vi "Begin.vi"(8 "error in":errorcluster) -> (0 "error out":errorcluster)   [LabVIEW 2015]
doc: "Called before other user functions, this VI is expected to open initial I/O refnums, load in file data, and do all program initialization. Notice that the <B>error out</B> terminal is simply used for data flow. Wiring it to other structures or subVIs ensures that this VI runs first."
uses:
  <vilib>/Rock Robotics/WPI/DriverStation/WPI_DriverStationRobotMode2.ctl
  <vilib>/Rock Robotics/WPI/Joystick/WPI_JoystickDeviceEnum.ctl
  <vilib>/Rock Robotics/WPI/Solenoid/WPI_SolenoidChannel.ctl
  <vilib>/Rock Robotics/WPI/CAN/TalonSRX/WPI_CANTalonSRX_BrakeOverride.ctl
  <vilib>/Rock Robotics/WPI/CAN/TalonSRX/WPI_CANTalonSRX_APIControlMode.ctl
  <vilib>/Rock Robotics/SystemInterfaces/DIO/FPGA_DIOChannel.ctl
  <vilib>/Rock Robotics/WPI/Camera/WPI_CameraWhite Balance Values.ctl
  <vilib>/Rock Robotics/WPI/Camera/WPI_CameraExposure Values.ctl
  Robot Global Data.vi
  <vilib>/Rock Robotics/WPI/Utilities/WPI_GetSetVariantRefNum.vi
  <vilib>/Rock Robotics/WPI/Solenoid/WPI_SolenoidOpenSingle.vi
  <vilib>/Rock Robotics/WPI/MotorControl/WPI_MotorControlOpenCANTalonSRX.vi
  <vilib>/Rock Robotics/SystemInterfaces/DIO/FPGA_DIOPWMChannel.ctl
  <vilib>/Rock Robotics/Network Tables/NT Write String Array.vi
  <vilib>/Rock Robotics/WPI/Counter/WPI_CounterDigitalInputToDigitalSource.vi
  <vilib>/Rock Robotics/WPI/RobotDrive/WPI_RobotDriveOpen2MotorWithTalon.vi
  <vilib>/Rock Robotics/WPI/SafetyOutput/WPI_SafetyOutputConfigMenu.ctl
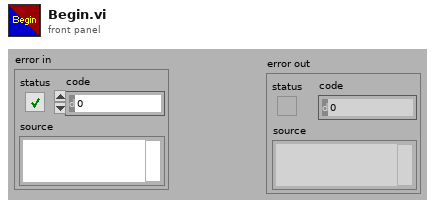
[diagram p1: front panel]
types:
  T1 = typedef "WPI_CANTalonSRX_BrakeOverride.ctl" = enum8{"No Override", "Override to Coast", "Override to Brake"}
  T2 = typedef "FPGA_DIOChannel.ctl" = enum8{"DIO 0", "DIO 1", "DIO 2", "DIO 3", "DIO 4", "DIO 5", "DIO 6", "DIO 7", "DIO 8", "DIO 9", "DIO MXP 0", "DIO MXP 1", "DIO MXP 2", "DIO MXP 3", "DIO MXP 4", "DIO MXP 5", "DIO MXP 6", "DIO MXP 7", "DIO MXP 8", "DIO MXP 9", "DIO MXP 10", "DIO MXP 11", "DIO MXP 12", "DIO MXP 13", "DIO MXP 14", "DIO MXP 15", "Invalid"}
  T3 = typedef "WPI_JoystickDeviceEnum.ctl" = enum16{"USB 0", "USB 1", "USB 2", "USB 3", "USB 4", "USB 5"}
  T4 = typedef "WPI_SolenoidChannel.ctl" = enum8{"Solenoid 0", "Solenoid 1", "Solenoid 2", "Solenoid 3", "Solenoid 4", "Solenoid 5", "Solenoid 6", "Solenoid 7", "Invalid"}
  T5 = typedef "WPI_CANTalonSRX_APIControlMode.ctl" = enum8{"Percent VBus", "Speed", "Position", "Slave", "Unchanged / Invalid", "Voltage Compensation", "Current", "Motion Profile"}
  T6 = typedef "WPI_DriverStationRobotMode2.ctl" = enum16{"Autonomous Disabled", "Autonomous Enabled", "Teleop Disabled", "Teleop Enabled", "Disconnected", "Finish", "Test Disabled", "Test Enabled", "Emergency Stopped"}
  T7 = typedef "WPI_CameraExposure Values.ctl" = enum16{"Auto", "Flicker-free 50 Hz", "Flicker-free 60 Hz", "Hold current", "Custom"}
  T8 = typedef "WPI_CameraWhite Balance Values.ctl" = enum16{"Auto", "Fixed indoor", "Fixed outdoor 1", "Fixed outdoor 2", "Fixed fluorescent 1", "Fixed fluorescent 2", "Hold current", "Custom"}
  T9 = typedef "WPI_CameraDevRef.ctl" = cluster{"Camera Address":string, "CameraStatus":errorcluster}
  T10 = typedef "WPI_DigitalInputDevRef.ctl" = cluster{"DevStatus":errorcluster, "DIO Channel":T2}
  T11 = typedef "FPGA_CounterEncoderSourceConvertionLVSourceType.ctl" = cluster{"DevStatus":errorcluster, "AnalogTriggerMode?":bool, "DigitalMode":cluster{"DIO Channel":T12}, "AnalogTriggerMode":cluster{"AnalogTriggerIndex":T13, "OutputType":T14}}
  T12 = typedef "FPGA_DIODigitalSourceChannel.ctl" = enum8{"DIO 0", "DIO 1", "DIO 2", "DIO 3", "DIO 4", "DIO 5", "DIO 6", "DIO 7", "DIO 8", "DIO 9", "DIO MXP 0", "DIO MXP 1", "DIO MXP 2", "DIO MXP 3", "DIO MXP 4", "DIO MXP 5", "DIO MXP 6", "DIO MXP 7", "DIO MXP 8", "DIO MXP 9", "DIO MXP 10", "DIO MXP 11", "DIO MXP 12", "DIO MXP 13", "DIO MXP 14", "DIO MXP 15", "Disabled"}
  T13 = typedef "FPGA_AnalogTriggerIndex.ctl" = enum8{"Trig 0", "Trig 1", "Trig 2", "Trig 3", "Trig 4", "Trig 5", "Trig 6", "Trig 7", "Invalid"}
  T14 = typedef "FPGA_AnalogTriggerOutType.ctl" = enum16{"InWindow", "TriggerState", "Rising", "Falling"}
  T15 = typedef "WPI_EncoderDevRef.ctl" = cluster{"DevStatus":errorcluster, "EncoderIndex":T16, "CounterIndex":T17, "DistancePerCount":dbl, "Decoding Type":T18}
  T16 = typedef "FPGA_EncoderIdx.ctl" = enum8{"Enc 0", "Enc 1", "Enc 2", "Enc 3", "Enc 4", "Enc 5", "Enc 6", "Enc 7", "Invalid"}
  T17 = typedef "FPGA_CounterCtrSystemIndex.ctl" = enum8{"Ctr 0", "Ctr 1", "Ctr 2", "Ctr 3", "Ctr 4", "Ctr 5", "Ctr 6", "Ctr 7", "Invalid"}
  T18 = typedef "WPI_EncoderType.ctl" = enum16{"1x", "2x", "4x"}
  T19 = typedef "WPI_SafetyOutputConfigMenu.ctl" = enum16{"Enable", "Disable"}
  T20 = typedef "FPGA_DIOPWMChannel.ctl" = enum8{"PWM 0", "PWM 1", "PWM 2", "PWM 3", "PWM 4", "PWM 5", "PWM 6", "PWM 7", "PWM 8", "PWM 9", "PWM MXP 0", "PWM MXP 1", "PWM MXP 2", "PWM MXP 3", "PWM MXP 4", "PWM MXP 5", "PWM MXP 6", "PWM MXP 7", "PWM MXP 8", "PWM MXP 9", "Invalid"}
  T21 = typedef "WPI_RobotDriveDevRef.ctl" = cluster{"DevStatus":errorcluster, "Motors[]":T22[], "Square Inputs":bool, "Max Output":dbl}
  T22 = typedef "WPI_MotorControlDeviceRef.ctl" = cluster{"DeviceStatus":errorcluster, "Type":T23, "PWM":cluster{"PWM Channel":T20, "DeadBand":T24}, "CAN":cluster{"Device Number":u8, "Control Mode":T25, "Semaphore":T26, "Max Vout":dbl, "TalonSRX Control Mode":T5}, "Invert":bool}
  T23 = typedef "WPI_MotorControlType.ctl" = enum16{"PWM", "CAN", "CANTalonSRX"}
  T24 = typedef "WPI_PWMDeadband.ctl" = cluster{"Name":string, "maxPositivePwm":i32, "minPositivePwm":i32, "centerPwm":i32, "maxNegativePwm":i32, "minNegativePwm":i32, "angularRange":u16}
  T25 = typedef "WPI_CANJaguar_ControlMode.ctl" = enum8{"Percent VBus", "Current", "Speed", "Position", "Voltage"}
  T26 = typedef "Semaphore RefNum" = refnum<k1>
  T27 = typedef "WPI_SolenoidDevRef.ctl" = cluster{"DevStatus":errorcluster, "Pneumatics Control Module":u8, "Forward Solenoid Channel":T4, "Reverse Solenoid Channel":T4}
  T28 = typedef "WPI_CompressorDevRef.ctl" = cluster{"DevStatus":errorcluster, "Pneumatics Control Module":u8}
  T29 = typedef "WPI_JoystickDevRef.ctl" = cluster{"Device":T3}
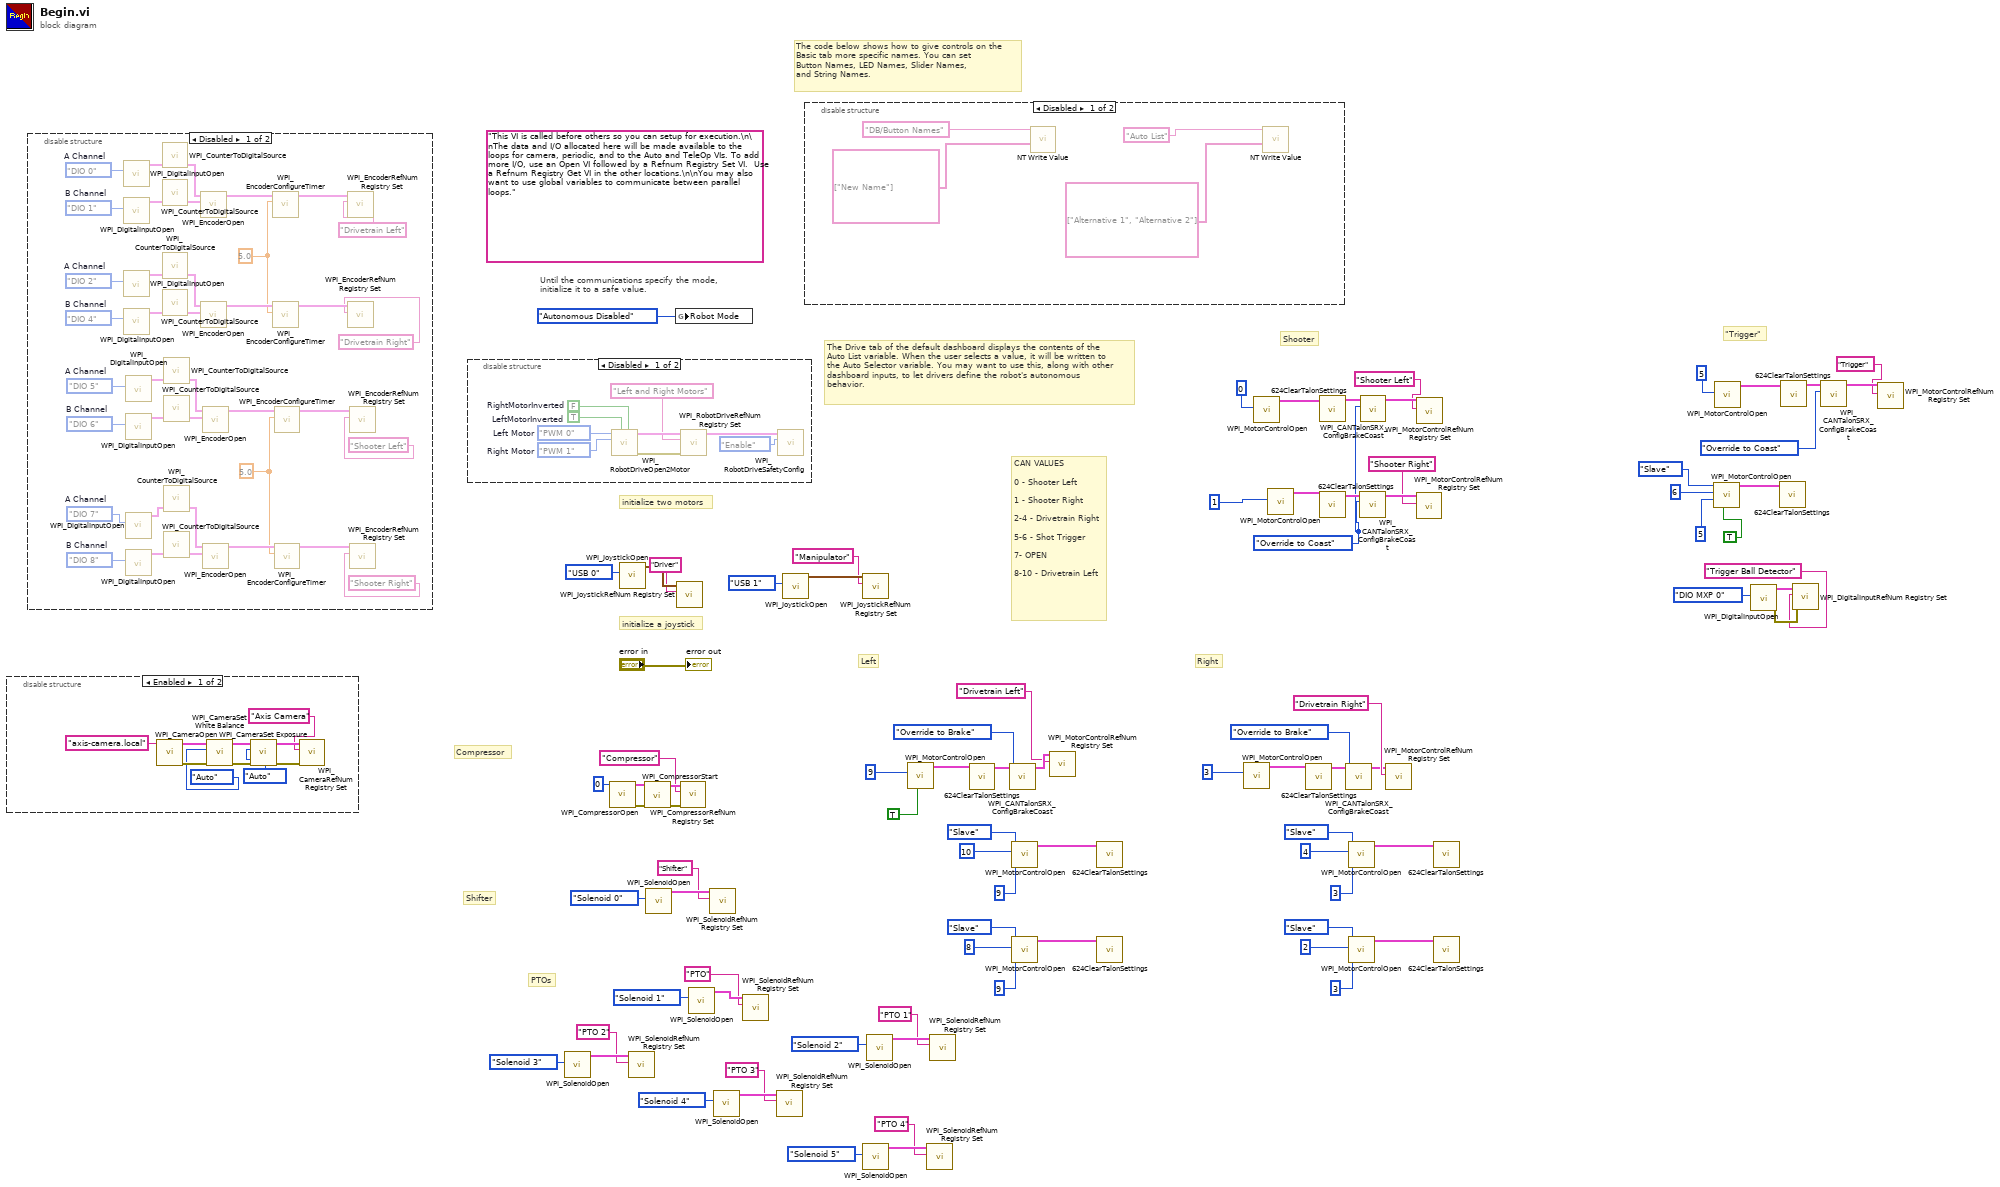
[diagram p0: block diagram]
diagram:
  w42 = WPI_CANTalonSRX_BrakeOverride."Override to Coast" ("Brake / Coast Mode")
  (unwired) "This VI is called before others so you can setup for execution.\n\nThe data and I/O allocated here will be made available to the loops for camera, periodic, and to the Auto and TeleOp VIs. To add more I/O, use an Open VI followed by a Refnum Registry Set VI.  Use a Refnum Registry Get VI in the other locations.\n\nYou may also want to use global variables to communicate between parallel loops."
  # "\"Trigger\""
  # "CAN VALUES\n\n0 - Shooter Left\n\n1 - Shooter Right\n\n2-4 - Drivetrain Right\n\n5-6 - Shot Trigger\n\n7- OPEN\n\n8-10 - Drivetrain Left"
  # "PTOs"
  # "Shooter"
  # "Left"
  # "Right"
  # "Shifter"
  # "Compressor"
  # "The Drive tab of the default dashboard displays the contents of the\nAuto List variable. When the user selects a value, it will be written to\nthe Auto Selector variable. You may want to use this, along with other\ndashboard inputs, to let drivers define the robot's autonomous\nbehavior."
  # "The code below shows how to give controls on the\nBasic tab more specific names. You can set\nButton Names, LED Names, Slider Names,\nand String Names."
  # "initialize a joystick"
  # "Until the communications specify the mode,\ninitialize it to a safe value."
  # "initialize two motors"
  n1 = disable-structure shown="Enabled" {
    frame Enabled {
      n2 = call <vilib>:"WPI_CameraOpen.vi"("Camera Address"="axis-camera.local") -> ("error out"=w93:errorcluster, "CameraDevRef"=w92:T9)  [unwired: 9 in]
      n3 = call <vilib>:"WPI_CameraSet White Balance.vi"("error in (no error)"=w93, "White Balance"=WPI_CameraWhite_Balance_Values."Auto", "CameraDevRef"=w92) -> ("error out"=w95:errorcluster, "CameraDevRef Out"=w94:T9)  [unwired: 7 in]
      n4 = call <vilib>:"WPI_CameraSet Exposure.vi"("error in (no error)"=w95, "Exposure"=WPI_CameraExposure_Values."Auto", "CameraDevRef"=w94) -> ("error out"=w97:errorcluster, "CameraDevRef Out"=w96:T9)  [unwired: 7 in]
      n5 = call <vilib>:"WPI_CameraRefNum Registry Set.vi"("error in (no error)"=w97, "refnum name"="Axis Camera", "CameraDevRef"=w96) -> ()  [unwired: 7 in, 2 out]
    }
    frame Disabled {
    }
  }
  n6 = disable-structure shown="Disabled" {
    frame Disabled {
      w100 = FPGA_DIOChannel."DIO 0"  # A Channel
      w103 = FPGA_DIOChannel."DIO 1"  # B Channel
      w108 = 5.0 ("Minimum Rate")
      w109 = FPGA_DIOChannel."DIO 2"  # A Channel
      w112 = FPGA_DIOChannel."DIO 4"  # B Channel
      w119 = FPGA_DIOChannel."DIO 6"  # B Channel
      w122 = FPGA_DIOChannel."DIO 5"  # A Channel
      w127 = 5.0 ("Minimum Rate")
      w128 = FPGA_DIOChannel."DIO 8"  # B Channel
      w131 = FPGA_DIOChannel."DIO 7"  # A Channel
      n7 = call <vilib>:"WPI_DigitalInputOpen.vi"("DIO Channel"=w100) -> ("DigitalInputDevRef"=w101:T10)  [unwired: 1 in, 9 out]
      n8 = call <vilib>:"WPI_DigitalInputOpen.vi"("DIO Channel"=w103) -> ("DigitalInputDevRef"=w104:T10)  [unwired: 1 in, 9 out]
      n9 = call <vilib>:"WPI_DigitalInputOpen.vi"("DIO Channel"=w109) -> ("DigitalInputDevRef"=w110:T10)  [unwired: 1 in, 9 out]
      n10 = call <vilib>:"WPI_DigitalInputOpen.vi"("DIO Channel"=w112) -> ("DigitalInputDevRef"=w113:T10)  [unwired: 1 in, 9 out]
      n11 = call <vilib>:"WPI_DigitalInputOpen.vi"("DIO Channel"=w122) -> ("DigitalInputDevRef"=w123:T10)  [unwired: 1 in, 9 out]
      n12 = call <vilib>:"WPI_DigitalInputOpen.vi"("DIO Channel"=w119) -> ("DigitalInputDevRef"=w120:T10)  [unwired: 1 in, 9 out]
      n13 = call <vilib>:"WPI_DigitalInputOpen.vi"("DIO Channel"=w131) -> ("DigitalInputDevRef"=w132:T10)  [unwired: 1 in, 9 out]
      n14 = call <vilib>:"WPI_DigitalInputOpen.vi"("DIO Channel"=w128) -> ("DigitalInputDevRef"=w129:T10)  [unwired: 1 in, 9 out]
      n15 = call-poly <vilib>:"WPI_CounterToDigitalSource.vi"("DigitalInputDevRef"=w101) -> ("Digital Source"=w102:T11)  [unwired: 6 out]
      n16 = call-poly <vilib>:"WPI_CounterToDigitalSource.vi"("DigitalInputDevRef"=w104) -> ("Digital Source"=w105:T11)  [unwired: 6 out]
      n17 = call-poly <vilib>:"WPI_CounterToDigitalSource.vi"("DigitalInputDevRef"=w110) -> ("Digital Source"=w111:T11)  [unwired: 6 out]
      n18 = call-poly <vilib>:"WPI_CounterToDigitalSource.vi"("DigitalInputDevRef"=w113) -> ("Digital Source"=w114:T11)  [unwired: 6 out]
      n19 = call-poly <vilib>:"WPI_CounterToDigitalSource.vi"("DigitalInputDevRef"=w123) -> ("Digital Source"=w124:T11)  [unwired: 6 out]
      n20 = call-poly <vilib>:"WPI_CounterToDigitalSource.vi"("DigitalInputDevRef"=w120) -> ("Digital Source"=w121:T11)  [unwired: 6 out]
      n21 = call-poly <vilib>:"WPI_CounterToDigitalSource.vi"("DigitalInputDevRef"=w132) -> ("Digital Source"=w133:T11)  [unwired: 6 out]
      n22 = call-poly <vilib>:"WPI_CounterToDigitalSource.vi"("DigitalInputDevRef"=w129) -> ("Digital Source"=w130:T11)  [unwired: 6 out]
      n23 = call <vilib>:"WPI_EncoderOpen.vi"("BSource"=w105, "ASource"=w102) -> ("EncoderDevRef"=w106:T15)  [unwired: 6 in, 3 out]
      n24 = call <vilib>:"WPI_EncoderOpen.vi"("BSource"=w114, "ASource"=w111) -> ("EncoderDevRef"=w115:T15)  [unwired: 6 in, 3 out]
      n25 = call <vilib>:"WPI_EncoderOpen.vi"("BSource"=w121, "ASource"=w124) -> ("EncoderDevRef"=w125:T15)  [unwired: 6 in, 3 out]
      n26 = call <vilib>:"WPI_EncoderOpen.vi"("BSource"=w130, "ASource"=w133) -> ("EncoderDevRef"=w134:T15)  [unwired: 6 in, 3 out]
      n27 = call <vilib>:"WPI_EncoderConfigureTimer.vi"("Minimum Rate"=w108, "EncoderDevRef"=w106) -> ("EncoderDevRef"=w107:T15)  [unwired: 8 in, 1 out]
      n28 = call <vilib>:"WPI_EncoderConfigureTimer.vi"("Minimum Rate"=w108, "EncoderDevRef"=w115) -> ("EncoderDevRef"=w116:T15)  [unwired: 8 in, 1 out]
      n29 = call <vilib>:"WPI_EncoderConfigureTimer.vi"("Minimum Rate"=w127, "EncoderDevRef"=w125) -> ("EncoderDevRef"=w126:T15)  [unwired: 8 in, 1 out]
      n30 = call <vilib>:"WPI_EncoderConfigureTimer.vi"("Minimum Rate"=w127, "EncoderDevRef"=w134) -> ("EncoderDevRef"=w135:T15)  [unwired: 8 in, 1 out]
      n31 = call <vilib>:"WPI_EncoderRefNum Registry Set.vi"("refnum name"="Drivetrain Left", "EncoderDevRef"=w107) -> ()  [unwired: 8 in, 2 out]
      n32 = call <vilib>:"WPI_EncoderRefNum Registry Set.vi"("refnum name"="Drivetrain Right", "EncoderDevRef"=w116) -> ()  [unwired: 8 in, 2 out]
      n33 = call <vilib>:"WPI_EncoderRefNum Registry Set.vi"("refnum name"="Shooter Left", "EncoderDevRef"=w126) -> ()  [unwired: 8 in, 2 out]
      n34 = call <vilib>:"WPI_EncoderRefNum Registry Set.vi"("refnum name"="Shooter Right", "EncoderDevRef"=w135) -> ()  [unwired: 8 in, 2 out]
    }
    frame Enabled {
    }
  }
  n35 = disable-structure shown="Disabled" {
    frame Disabled {
      w138 = FPGA_DIOPWMChannel."PWM 1"  # Right Motor
      w139 = TRUE  # LeftMotorInverted
      w140 = FPGA_DIOPWMChannel."PWM 0"  # Left Motor
      w141 = FALSE  # RightMotorInverted
      n36 = call-poly <vilib>:"WPI_RobotDriveOpen2Motor.vi"("Right Motor Inverted"=w141, "Left Motor Inverted"=w139, "Right Motor"=w138, "Left Motor"=w140) -> ("error out"=w143:errorcluster, "RobotDriveDevRef"=w142:T21)  [unwired: 1 in, 5 out]
      n37 = call <vilib>:"WPI_RobotDriveRefNum Registry Set.vi"("error in (no error)"=w143, "refnum name"="Left and Right Motors", "RobotDriveDevRef"=w142) -> ("RobotDriveDevRef"=w144:T21)  [unwired: 1 in, 7 out]
      n38 = call <vilib>:"WPI_RobotDriveSafetyConfig.vi"("mode"=WPI_SafetyOutputConfigMenu."Enable", "RobotDriveDevRef"=w144) -> ()  [unwired: 8 in, 2 out]
    }
    frame Enabled {
    }
  }
  n39 = call-poly <vilib>:"WPI_SolenoidOpen.vi"("Solenoid Channel"=WPI_SolenoidChannel."Solenoid 3") -> ("SolenoidDevRef"=w27:T27)  [unwired: 9 in, 1 out]
  n40 = call <vilib>:"WPI_CompressorOpen.vi"("Pneumatics Control Module (0)"=0) -> ("CompressorDevRef"=w82:T28, "error out"=w79:errorcluster)  [unwired: 13 in]
  n41 = call <vilib>:"WPI_JoystickOpen.vi"("JoystickDevice"=WPI_JoystickDeviceEnum."USB 0") -> ("JoystickDevRef"=w86:T29)  [unwired: 10 in]
  n42 = call <vilib>:"WPI_SolenoidRefNum Registry Set.vi"("refnum name"="PTO 2", "SolenoidDevRef"=w27) -> ()  [unwired: 8 in, 2 out]
  n43 = call <vilib>:"WPI_CompressorStart.vi"("error in (no error)"=w79, "CompressorDevRef"=w82) -> ("error out"=w78:errorcluster, "CompressorDevRef"=w81:T28)  [unwired: 8 in]
  n44 = call-poly <vilib>:"WPI_SolenoidOpen.vi"("Solenoid Channel"=WPI_SolenoidChannel."Solenoid 0") -> ("SolenoidDevRef"=w76:T27)  [unwired: 9 in, 1 out]
  n45 = global write "Robot Global Data.vi" "Robot Mode"(WPI_DriverStationRobotMode2."Autonomous Disabled" ("Robot Mode")) -> ()
  n46 = call <vilib>:"WPI_JoystickRefNum Registry Set.vi"("refnum name"="Driver", "JoystickDevRef"=w86) -> ()  [unwired: 8 in, 2 out]
  n47 = call <vilib>:"WPI_CompressorRefNum Registry Set.vi"("error in (no error)"=w78, "refnum name"="Compressor", "CompressorDevRef"=w81) -> ()  [unwired: 7 in, 2 out]
  n48 = call-poly <vilib>:"WPI_SolenoidOpen.vi"("Solenoid Channel"=WPI_SolenoidChannel."Solenoid 1") -> ("SolenoidDevRef"=w35:T27)  [unwired: 9 in, 1 out]
  n49 = call <vilib>:"WPI_SolenoidRefNum Registry Set.vi"("refnum name"="Shifter", "SolenoidDevRef"=w76) -> ()  [unwired: 8 in, 2 out]
  n50 = call-poly <vilib>:"WPI_SolenoidOpen.vi"("Solenoid Channel"=WPI_SolenoidChannel."Solenoid 4") -> ("SolenoidDevRef"=w30:T27)  [unwired: 9 in, 1 out]
  n51 = call <vilib>:"WPI_SolenoidRefNum Registry Set.vi"("refnum name"="PTO", "SolenoidDevRef"=w35) -> ()  [unwired: 8 in, 2 out]
  n52 = call <vilib>:"WPI_SolenoidRefNum Registry Set.vi"("refnum name"="PTO 3", "SolenoidDevRef"=w30) -> ()  [unwired: 8 in, 2 out]
  n53 = call <vilib>:"WPI_JoystickOpen.vi"("JoystickDevice"=WPI_JoystickDeviceEnum."USB 1") -> ("JoystickDevRef"=w21:T29)  [unwired: 10 in]
  n54 = disable-structure shown="Disabled" {
    frame Disabled {
      n55 = call-poly <vilib>:"NT Write Value.vi"("String Array"=string[] ["New Name"], "Name"="DB/Button Names") -> ()  [unwired: 9 in, 1 out]
      n56 = call-poly <vilib>:"NT Write Value.vi"("String Array"=string[] ["Alternative 1", "Alternative 2"], "Name"="Auto List") -> ()  [unwired: 9 in, 1 out]
    }
    frame Enabled {
    }
  }
  n57 = call <vilib>:"WPI_JoystickRefNum Registry Set.vi"("refnum name"="Manipulator", "JoystickDevRef"=w21) -> ()  [unwired: 8 in, 2 out]
  n58 = call-poly <vilib>:"WPI_SolenoidOpen.vi"("Solenoid Channel"=WPI_SolenoidChannel."Solenoid 5") -> ("SolenoidDevRef"=w24:T27)  [unwired: 9 in, 1 out]
  n59 = call-poly <vilib>:"WPI_SolenoidOpen.vi"("Solenoid Channel"=WPI_SolenoidChannel."Solenoid 2") -> ("SolenoidDevRef"=w33:T27)  [unwired: 9 in, 1 out]
  n60 = call-poly <vilib>:"WPI_MotorControlOpen.vi"("Invert"=TRUE, "Device Number"=9) -> ("MotorControlDeviceRef"=w50:T22)  [unwired: 8 in, 1 out]
  n61 = call <vilib>:"WPI_SolenoidRefNum Registry Set.vi"("refnum name"="PTO 4", "SolenoidDevRef"=w24) -> ()  [unwired: 8 in, 2 out]
  n62 = call <vilib>:"WPI_SolenoidRefNum Registry Set.vi"("refnum name"="PTO 1", "SolenoidDevRef"=w33) -> ()  [unwired: 8 in, 2 out]
  n63 = call "624ClearTalonSettings.vi"("CAN Talon SRX Ref Out"=w50) -> ("CAN Talon SRX Ref Out 2"=w51:T22)  [unwired: 10 in]
  n64 = call <vilib>:"WPI_CANTalonSRX_ConfigBrakeCoast.vi"("Brake / Coast Mode"=WPI_CANTalonSRX_BrakeOverride."Override to Brake", "CAN Talon SRX Ref"=w51) -> ("CAN Talon SRX Ref"=w52:T22)  [unwired: 8 in, 1 out]
  n65 = call-poly <vilib>:"WPI_MotorControlOpen.vi"("Master Device Number"=u8 9, "Device Number"=u8 10, "Control Mode"=WPI_CANTalonSRX_APIControlMode."Slave") -> ("MotorControlDeviceRef"=w56:T22)  [unwired: 7 in, 1 out]
  n66 = call-poly <vilib>:"WPI_MotorControlOpen.vi"("Master Device Number"=u8 9, "Device Number"=u8 8, "Control Mode"=WPI_CANTalonSRX_APIControlMode."Slave") -> ("MotorControlDeviceRef"=w57:T22)  [unwired: 7 in, 1 out]
  n67 = call <vilib>:"WPI_MotorControlRefNum Registry Set.vi"("refnum name"="Drivetrain Left", "MotorControlDevRef"=w52) -> ()  [unwired: 8 in, 2 out]
  n68 = call "624ClearTalonSettings.vi"("CAN Talon SRX Ref Out"=w56) -> ()  [unwired: 10 in, 1 out]
  n69 = call "624ClearTalonSettings.vi"("CAN Talon SRX Ref Out"=w57) -> ()  [unwired: 10 in, 1 out]
  n70 = call-poly <vilib>:"WPI_MotorControlOpen.vi"("Device Number"=3) -> ("MotorControlDeviceRef"=w71:T22)  [unwired: 9 in, 1 out]
  n71 = call-poly <vilib>:"WPI_MotorControlOpen.vi"("Device Number"=u8 0) -> ("MotorControlDeviceRef"=w39:T22)  [unwired: 9 in, 1 out]
  n72 = call-poly <vilib>:"WPI_MotorControlOpen.vi"("Device Number"=u8 1) -> ("MotorControlDeviceRef"=w44:T22)  [unwired: 9 in, 1 out]
  n73 = call "624ClearTalonSettings.vi"("CAN Talon SRX Ref Out"=w71) -> ("CAN Talon SRX Ref Out 2"=w70:T22)  [unwired: 10 in]
  n74 = call "624ClearTalonSettings.vi"("CAN Talon SRX Ref Out"=w44) -> ("CAN Talon SRX Ref Out 2"=w45:T22)  [unwired: 10 in]
  n75 = call "624ClearTalonSettings.vi"("CAN Talon SRX Ref Out"=w39) -> ("CAN Talon SRX Ref Out 2"=w40:T22)  [unwired: 10 in]
  n76 = call <vilib>:"WPI_CANTalonSRX_ConfigBrakeCoast.vi"("Brake / Coast Mode"=WPI_CANTalonSRX_BrakeOverride."Override to Brake", "CAN Talon SRX Ref"=w70) -> ("CAN Talon SRX Ref"=w69:T22)  [unwired: 8 in, 1 out]
  n77 = call-poly <vilib>:"WPI_MotorControlOpen.vi"("Master Device Number"=u8 3, "Device Number"=u8 4, "Control Mode"=WPI_CANTalonSRX_APIControlMode."Slave") -> ("MotorControlDeviceRef"=w65:T22)  [unwired: 7 in, 1 out]
  n78 = call-poly <vilib>:"WPI_MotorControlOpen.vi"("Master Device Number"=u8 3, "Device Number"=u8 2, "Control Mode"=WPI_CANTalonSRX_APIControlMode."Slave") -> ("MotorControlDeviceRef"=w64:T22)  [unwired: 7 in, 1 out]
  n79 = call <vilib>:"WPI_CANTalonSRX_ConfigBrakeCoast.vi"("Brake / Coast Mode"=w42, "CAN Talon SRX Ref"=w45) -> ("CAN Talon SRX Ref"=w46:T22)  [unwired: 8 in, 1 out]
  n80 = call <vilib>:"WPI_CANTalonSRX_ConfigBrakeCoast.vi"("Brake / Coast Mode"=w42, "CAN Talon SRX Ref"=w40) -> ("CAN Talon SRX Ref"=w41:T22)  [unwired: 8 in, 1 out]
  n81 = call <vilib>:"WPI_MotorControlRefNum Registry Set.vi"("refnum name"="Drivetrain Right", "MotorControlDevRef"=w69) -> ()  [unwired: 8 in, 2 out]
  n82 = call <vilib>:"WPI_MotorControlRefNum Registry Set.vi"("refnum name"="Shooter Right", "MotorControlDevRef"=w46) -> ()  [unwired: 8 in, 2 out]
  n83 = call <vilib>:"WPI_MotorControlRefNum Registry Set.vi"("refnum name"="Shooter Left", "MotorControlDevRef"=w41) -> ()  [unwired: 8 in, 2 out]
  n84 = call "624ClearTalonSettings.vi"("CAN Talon SRX Ref Out"=w65) -> ()  [unwired: 10 in, 1 out]
  n85 = call "624ClearTalonSettings.vi"("CAN Talon SRX Ref Out"=w64) -> ()  [unwired: 10 in, 1 out]
  n86 = call-poly <vilib>:"WPI_MotorControlOpen.vi"("Invert"=TRUE, "Master Device Number"=u8 5, "Device Number"=u8 6, "Control Mode"=WPI_CANTalonSRX_APIControlMode."Slave") -> ("MotorControlDeviceRef"=w7:T22)  [unwired: 6 in, 1 out]
  n87 = call-poly <vilib>:"WPI_MotorControlOpen.vi"("Device Number"=u8 5) -> ("MotorControlDeviceRef"=w10:T22)  [unwired: 9 in, 1 out]
  n88 = call <vilib>:"WPI_DigitalInputOpen.vi"("DIO Channel"=FPGA_DIOChannel."DIO MXP 0") -> ("error out"=w18:errorcluster, "DigitalInputDevRef"=w17:T10)  [unwired: 9 in]
  n89 = call "624ClearTalonSettings.vi"("CAN Talon SRX Ref Out"=w7) -> ()  [unwired: 10 in, 1 out]
  n90 = call "624ClearTalonSettings.vi"("CAN Talon SRX Ref Out"=w10) -> ("CAN Talon SRX Ref Out 2"=w11:T22)  [unwired: 10 in]
  n91 = call <vilib>:"WPI_DigitalInputRefNum Registry Set.vi"("error in (no error)"=w18, "refnum name"="Trigger Ball Detector", "DigitalInputDevRef"=w17) -> ()  [unwired: 7 in, 2 out]
  n92 = call <vilib>:"WPI_CANTalonSRX_ConfigBrakeCoast.vi"("Brake / Coast Mode"=WPI_CANTalonSRX_BrakeOverride."Override to Coast", "CAN Talon SRX Ref"=w11) -> ("CAN Talon SRX Ref"=w12:T22)  [unwired: 8 in, 1 out]
  n93 = call <vilib>:"WPI_MotorControlRefNum Registry Set.vi"("refnum name"="Trigger", "MotorControlDevRef"=w12) -> ()  [unwired: 8 in, 2 out]
  "error out" <- "error in"
